vi "Reception.vi"(0 "entrée d'erreur (pas d'erreur)":errorcluster, 1 "Nom de ressource VISA":refnum<visa-resource-name>) -> (2 "Sortie d'erreur":errorcluster caption="entrée d'erreur (pas d'erreur)", 3 "Checksum OK?":bool=TRUE, 4 "Data":sgl format="%.2f", 5 "ID byte":i32)   [LabVIEW 2010]
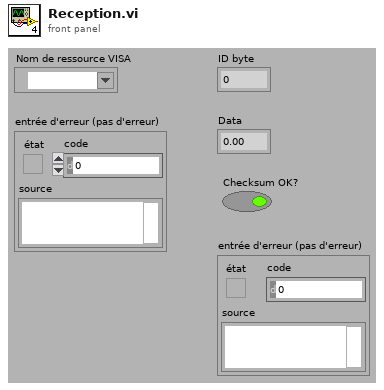
[diagram p1: front panel]
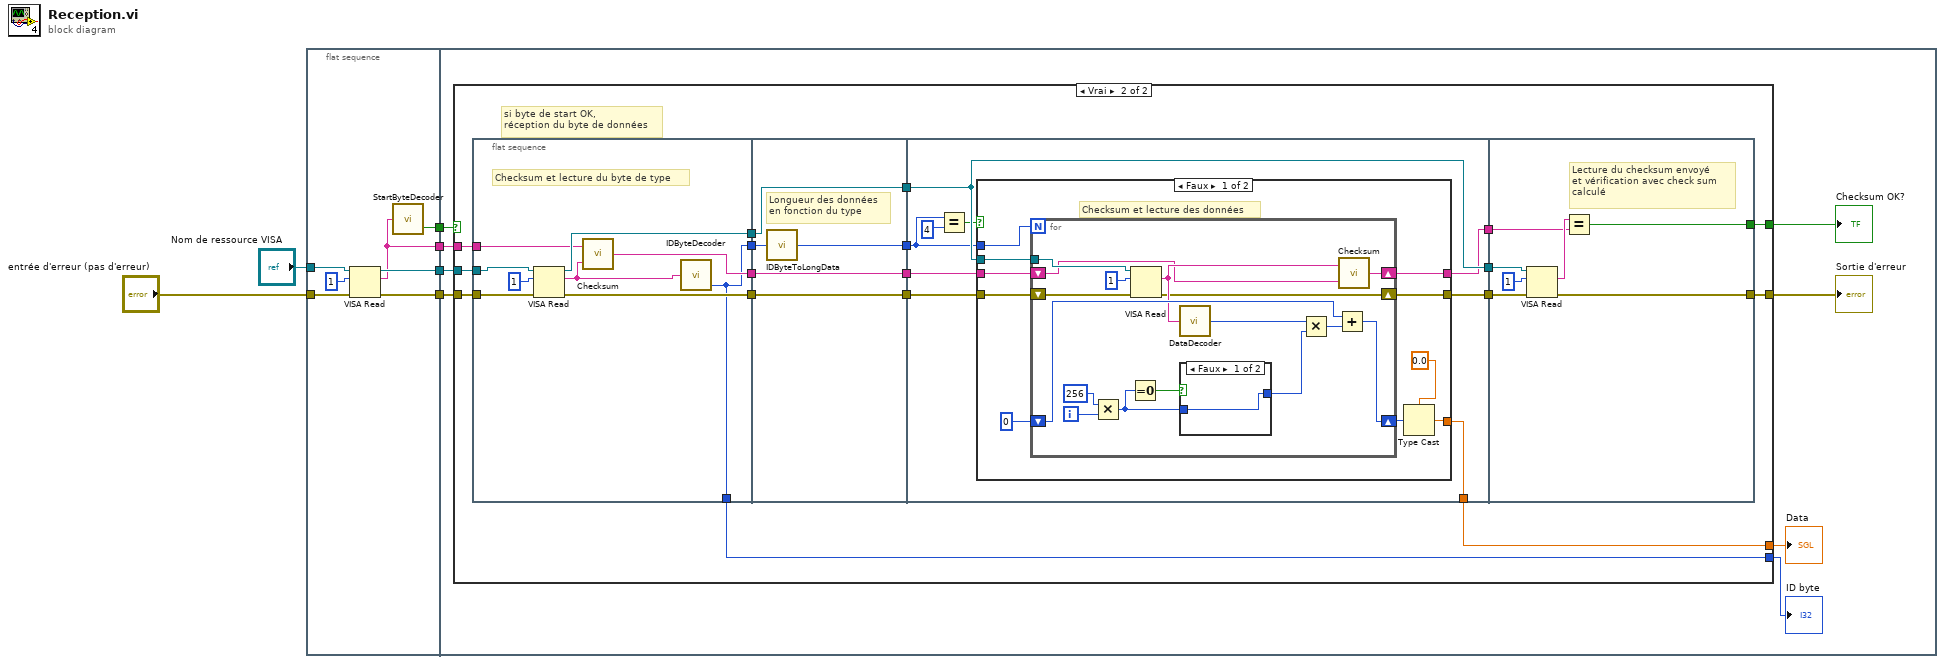
[diagram p0: block diagram]
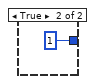
[diagram p3: hidden frame]
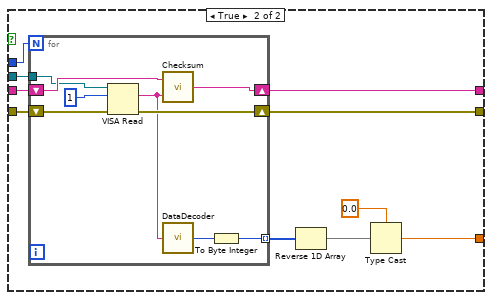
[diagram p4: hidden frame]
diagram:
  n1 = flat-sequence {
    tunnel: "Nom de ressource VISA" -> [w13]
    tunnel: "entrée d'erreur (pas d'erreur)" -> [w11]
    tunnel: [w10] -> w6
    tunnel: [w9] -> w5
    tunnel: [w8] -> w4
    tunnel: [w7] -> w3
    tunnel: w6 -> [w21]
    tunnel: w5 -> [w20]
    tunnel: w4 -> [w19]
    tunnel: w3 -> [w18]
    frame #0 {
      n2 = VISA Read(VISA resource name=w13, byte count=u32 1 ("nombre d'octets"), error in (no error)=w11) -> (VISA resource name out=w9:refnum<visa-resource-name>, read buffer=w7:string, error out=w8:errorcluster)  [unwired: 1 out]
      n3 = call "StartByteDecoder.vi"("byte1"=w7) -> ("Byte Start ?"=w10:bool)  [unwired: 1 in]
    }
    frame #1 {
      n4 = case shown="Vrai" w21 {
        tunnel: w20 -> [_ w40]
        tunnel: w19 -> [w22 w39]
        tunnel: w18 -> [_ w32]
        tunnel: [_ w26] -> w17
        tunnel: [_ w25] -> w16
        tunnel: [_ w24] -> w15
        tunnel: [w22 w23] -> w14
        frame False {
        }
        frame True {
          # "si byte de start OK,\nréception du byte de données"
          n5 = flat-sequence {
            tunnel: w40 -> [w49]
            tunnel: w39 -> [w47]
            tunnel: [w41] -> w38
            tunnel: [w46] -> w36
            tunnel: [w45] -> w34
            tunnel: w32 -> [w43]
            tunnel: [w42] -> w30
            tunnel: [w41] -> w26
            tunnel: w38 -> [w54]
            tunnel: [w53] -> w37
            tunnel: w36 -> [w52]
            tunnel: [w52] -> w35
            tunnel: w34 -> [w51]
            tunnel: [w51] -> w33
            tunnel: [w50] -> w31
            tunnel: w30 -> [w50]
            tunnel: w37 -> [w57]
            tunnel: w35 -> [w61]
            tunnel: w33 -> [w63]
            tunnel: w31 -> [w62]
            tunnel: [w61] -> w29
            tunnel: [w60] -> w28
            tunnel: [w59] -> w27
            tunnel: [w58] -> w25
            tunnel: w29 -> [w116]
            tunnel: w28 -> [w115]
            tunnel: w27 -> [w113]
            tunnel: [w112] -> w24
            tunnel: [w111] -> w23
            frame #0 {
              # "Checksum et lecture du byte de type"
              n6 = VISA Read(VISA resource name=w49, byte count=u32 1 ("nombre d'octets"), error in (no error)=w47) -> (VISA resource name out=w46:refnum<visa-resource-name>, read buffer=w44:string, error out=w45:errorcluster)  [unwired: 1 out]
              n7 = call "Checksum.vi"("Byte2"=w44, "Byte1"=w43) -> ("chaîne"=w42:string)
              n8 = call "IDByteDecoder.vi"("byte1"=w44) -> ("Type de donnee (ID)"=w41:i32)  [unwired: 2 out]
            }
            frame #1 {
              # "Longueur des données\nen fonction du type"
              n9 = call "IDByteToLongData.vi"("ID Byte"=w54) -> ("Data Long"=w53:i32)
            }
            frame #2 {
              n10 = Equal?(x=w57, y=4) -> (x = y?=w55:bool)
              n11 = case shown="Faux" w55 {
                tunnel: w63 -> [w73 w97]
                tunnel: w57 -> [w72 w101]
                tunnel: w62 -> [w70 w100]
                tunnel: w61 -> [w69 w99]
                tunnel: [w68 w96] -> w60
                tunnel: [w67 w98] -> w59
                tunnel: [w64 w94] -> w58
                frame False {
                  # "Checksum et lecture des données"
                  n12 = for {
                    N: w72 -> [_]
                    tunnel: w69 -> [w89]
                    shift-right: [w81] -> w65
                    shift-left: 0 -> [w82]
                    shift-right: [w78] -> w67
                    shift-left: w70 -> [w79]
                    shift-right: [w77] -> w68
                    shift-left: w73 -> [w88]
                    i -> [w86]
                    n13 = Multiply(x=256, y=w86) -> (x*y=w74:i32)
                    n14 = Equal To 0?(x=w74) -> (x = 0?=w76:bool)
                    n15 = VISA Read(VISA resource name=w89, byte count=u32 1 ("nombre d'octets"), error in (no error)=w88) -> (read buffer=w80:string, error out=w77:errorcluster)  [unwired: 2 out]
                    n16 = call "DataDecoder.vi"("byte1"=w80) -> ("Data"=w84:i32)
                    n17 = case shown="Faux" w76 {
                      tunnel: [w90 1 ("x")] -> w75
                      tunnel: w74 -> [w90 _]
                      frame False {
                      }
                      frame True {
                      }
                    }
                    n18 = Multiply(x=w84, y=w75) -> (x*y=w83:i32)
                    n19 = Add(x=w82, y=w83) -> (x+y=w81:i32)
                    n20 = call "Checksum.vi"("Byte2"=w79, "Byte1"=w80) -> ("chaîne"=w78:string)
                  }
                  n21 = Type Cast(type=sgl 0.0, x=w65) -> (*(type *) &x=w64:sgl)
                }
                frame True {
                  n22 = for {
                    N: w101 -> [_]
                    shift-right: [w110] -> w98
                    shift-left: w100 -> [w109]
                    tunnel: w99 -> [w108]
                    shift-right: [w105] -> w96
                    shift-left: w97 -> [w106]
                    tunnel: [w102] -> w93 mode=indexing
                    n23 = VISA Read(VISA resource name=w108, byte count=u32 1 ("nombre d'octets"), error in (no error)=w106) -> (read buffer=w104:string, error out=w105:errorcluster)  [unwired: 2 out]
                    n24 = call "Checksum.vi"("Byte2"=w104, "Byte1"=w109) -> ("chaîne"=w110:string)
                    n25 = call "DataDecoder.vi"("byte1"=w104) -> ("Data"=w103:i32)
                    n26 = To Byte Integer(number=w103) -> (8bit integer=w102:i8)
                  }
                  n27 = Reverse 1D Array(array=w93) -> (reversed array=w92:i8[])
                  n28 = Type Cast(type=sgl 0.0, x=w92) -> (*(type *) &x=w94:sgl)
                }
              }
            }
            frame #3 {
              # "Lecture du checksum envoyé\net vérification avec check sum \ncalculé"
              n29 = VISA Read(VISA resource name=w116, byte count=u32 1 ("nombre d'octets"), error in (no error)=w115) -> (read buffer=w114:string, error out=w111:errorcluster)  [unwired: 2 out]
              n30 = Equal?(x=w114, y=w113) -> (x = y?=w112:bool)
            }
          }
        }
      }
      "ID byte" <- w17
      "Data" <- w16
      "Checksum OK?" <- w15
      "Sortie d'erreur" <- w14
    }
  }
